vi "PictureHandler.vi"(8 "error in (no error)":errorcluster, 10 "Use static images? (t)":bool=TRUE, 11 "Picture":T1) -> (0 "error out":errorcluster, 3 "image data":T2)   [LabVIEW 2022 SP3, in "lv-attitudecontrol.lvlib"]
uses:
  lv-attitudecontrol.lvlib
  <vilib>/picture/picture.llb/imagedata.ctl
  Controls/PictureTypes.ctl
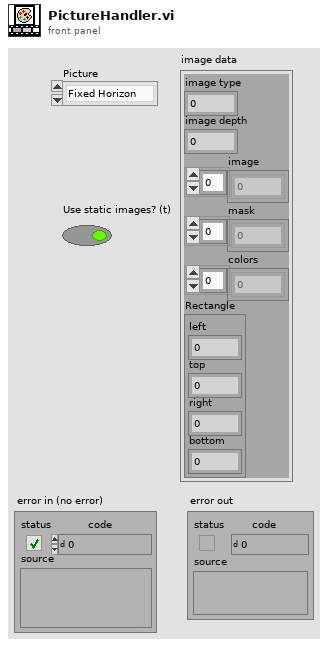
[diagram p1: front panel]
types:
  T1 = typedef "lv-attitudecontrol.lvlib/PictureTypes.ctl" = enum16{"Fixed Horizon", "Altitude Lines", "Dial"}
  T2 = typedef "imagedata.ctl" = cluster{"image type":i32, "image depth":i32, "image":u8[], "mask":u8[], "colors":u32[], "Rectangle":cluster{"left":i16, "top":i16, "right":i16, "bottom":i16}}
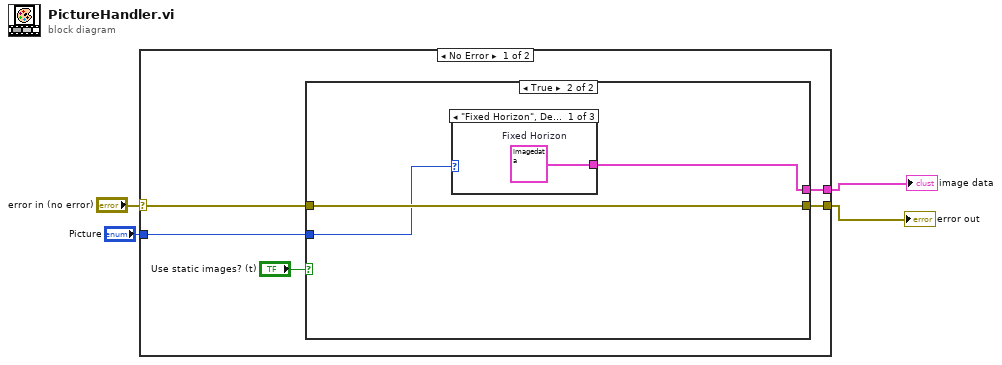
[diagram p0: block diagram]
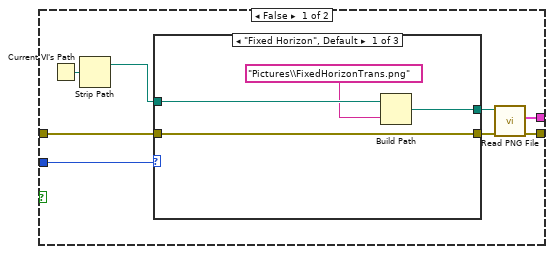
[diagram p2: hidden frame]
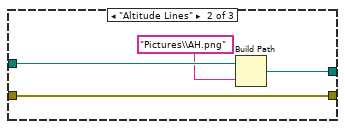
[diagram p3: hidden frame]
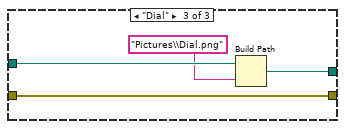
[diagram p4: hidden frame]
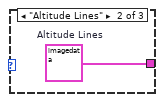
[diagram p5: hidden frame]
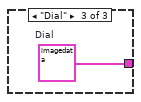
[diagram p6: hidden frame]
diagram:
  n1 = case shown="No Error" "error in (no error)" {
    selector: "error in (no error)" -> [w6 w36]
    tunnel: [w9 _] -> w4
    tunnel: [w8 w36] -> w3
    tunnel: "Picture" -> [w7 _]
    frame No Error {
      n2 = case shown="True" "Use static images? (t)" {
        tunnel: [w16 w31] -> w9
        tunnel: [w15 w32] -> w8
        tunnel: w7 -> [w14 w30]
        tunnel: w6 -> [w11 w32]
        frame False {
          n3 = Current VI's Path() -> (path=w13:path)
          n4 = Strip Path(path=w13) -> (stripped path=w12:path)  [unwired: 1 out]
          n5 = case shown="\"Fixed Horizon\", Default" w14 {
            tunnel: w12 -> [w21 w25 w29]
            tunnel: [w19 w23 w27] -> w17
            tunnel: w11 -> [w18 w22 w26]
            tunnel: [w18 w22 w26] -> w10
            frame "Fixed Horizon", Default {
              n6 = Build Path(base path=w21, name or relative path="Pictures\\FixedHorizonTrans.png") -> (appended path=w19:path)
            }
            frame "Altitude Lines" {
              n7 = Build Path(base path=w25, name or relative path="Pictures\\AH.png") -> (appended path=w23:path)
            }
            frame "Dial" {
              n8 = Build Path(base path=w29, name or relative path="Pictures\\Dial.png") -> (appended path=w27:path)
            }
          }
          n9 = call <vilib>:"Read PNG File.vi"("error in (no error)"=w10, "path to PNG file"=w17) -> ("error out"=w15:errorcluster, "image data"=w16:T2)  [unwired: 7 in, 1 out]
        }
        frame True {
          n10 = case shown="\"Fixed Horizon\", Default" w30 {
            tunnel: [w33 w34 w35] -> w31
            frame "Fixed Horizon", Default {
              w33 = T2 {"image type"=0, "image depth"=32, "image"=array[896808 elements], "mask"=array[28380 elements], "colors"=[], "Rectangle"={"left"=0, "top"=0, "right"=474, "bottom"=473}}  # Fixed Horizon
            }
            frame "Altitude Lines" {
              w34 = T2 {"image type"=0, "image depth"=32, "image"=array[922116 elements], "mask"=array[29302 elements], "colors"=[], "Rectangle"={"left"=0, "top"=0, "right"=771, "bottom"=299}}  # Altitude Lines
            }
            frame "Dial" {
              w35 = T2 {"image type"=0, "image depth"=32, "image"=array[1008016 elements], "mask"=array[32128 elements], "colors"=[], "Rectangle"={"left"=0, "top"=0, "right"=502, "bottom"=502}}  # Dial
            }
          }
        }
      }
    }
    frame Error {
    }
  }
  "image data" <- w4
  "error out" <- w3
